vi "example1.vi"() -> ()   [LabVIEW 2018]
uses:
  Commands.ctl
  LV-Julia_ZMQ-Roundtrip_lib.lvlib
panel:
  out "error now":errorcluster
  out "error out":errorcluster
  out "server response":string
  in  "data to send":string="hello"
  in  "stop":bool
  in  "milliseconds to wait":u32=1000
  in  "Julia ZMQ server file name":string="ZMQ-testserver2.jl"
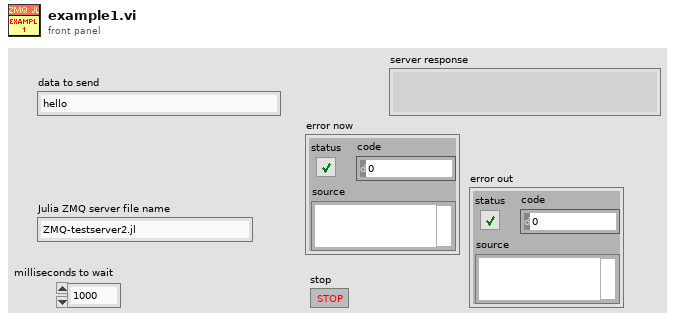
[diagram p1: front panel]
types:
  T1 = typedef "LV-Julia_ZMQ-Roundtrip_lib.lvlib/Commands.ctl" = enum16{"Start server", "Send request ", "Stop server", "Force clean-up"}
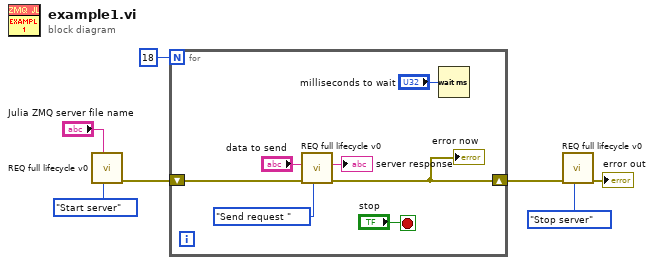
[diagram p0: block diagram]
diagram:
  n1 = call "REQ full lifecycle v0.vi"("command"=Commands."Start server", "Julia ZMQ server file name"="Julia ZMQ server file name") -> ("error out"=w5:errorcluster)  [unwired: 8 in, 1 out]
  n2 = for {
    N: 18 -> [_]
    shift-right: [w11] -> w4
    shift-left: w5 -> [w13]
    stop <- "stop" stop-if-true
    n3 = call "REQ full lifecycle v0.vi"("command"=Commands."Send request ", "error in"=w13, "data to send"="data to send") -> ("error out"=w11:errorcluster, "server response"=→"server response":string)  [unwired: 7 in]
    "error now" <- w11
    n4 = Wait (ms)(milliseconds to wait="milliseconds to wait") -> ()  [unwired: 1 out]
  }
  n5 = call "REQ full lifecycle v0.vi"("command"=Commands."Stop server", "error in"=w4) -> ("error out"=→"error out":errorcluster)  [unwired: 8 in, 1 out]
